vi "行号.vi"(8 "错误输入（无错误）":errorcluster, 9 "外观属性":T1={"大小"=15, "粗体"=FALSE, "下划线"=FALSE, "斜体"=FALSE, "背景色"=0, "前景色"=16448250, "Font"=""}, 11 "Scintilla":refnum<k24>) -> (0 "错误输出":errorcluster, 3 "引用输出":refnum<k24>)   [LabVIEW 2020]
uses:
  D:/SuperPython-master/ScintillaNET.dll
  ScintillaNET.dll
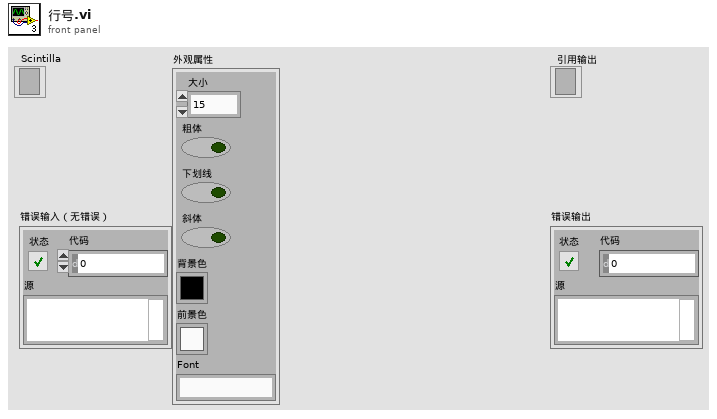
[diagram p1: front panel]
types:
  T1 = cluster{"大小":i32, "粗体":bool, "下划线":bool, "斜体":bool, "背景色":u32, "前景色":u32, "Font":string}
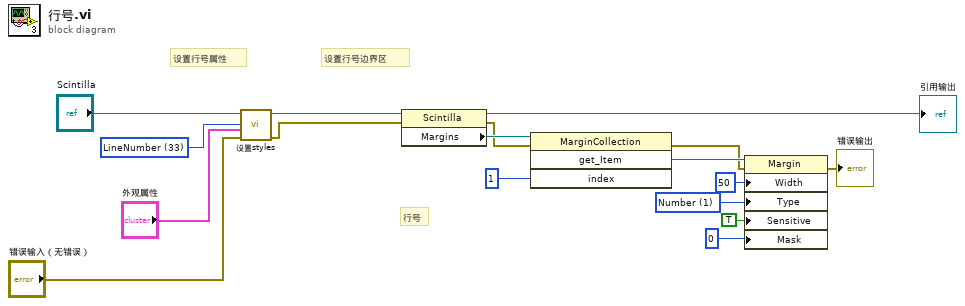
[diagram p0: block diagram]
diagram:
  w12 = 1 items=["Symbol", "Number", "BackColor", "ForeColor", "Text", "RightText", "Color"] ("Type")
  w8 = 33 items=["Default"=32, "LineNumber"=33, "BraceLight"=34, "BraceBad"=35, "IndentGuide"=37, "CallTip"=38, "FoldDisaplayText"=39] ("设置项")
  # "行号"
  # "设置行号边界区"
  # "设置行号属性"
  n1 = call "设置styles.vi"("错误输入（无错误）"="错误输入（无错误）", "外观属性"="外观属性", "设置项"=w8, "Scintilla"="Scintilla") -> ("错误输出"=w2:errorcluster, "Scintilla"=w3:refnum<k24>)  [unwired: 6 in]
  n2 = property class="Scintilla"(reference=w3, error in=w2) -> (reference out=→"引用输出":refnum<k24>, error out=w7:errorcluster, "Margins"=w17:refnum<k24>)
  n3 = invoke class="MarginCollection" method="get_Item"(reference=w17, error in=w7, "index"=1) -> (error out=w6:errorcluster, "get_Item"=w15:refnum<k24>)  [unwired: 1 in, 2 out]
  n4 = property class="Margin"(reference=w15, error in=w6, "Width"=50, "Type"=w12, "Sensitive"=TRUE, "Mask"=u32 0) -> (error out=→"错误输出":errorcluster)  [unwired: 1 out]
